vi "getServerCapabilities.vi"(8 "error in (no error)":errorcluster, 11 "IDeviceInfo in":refnum<class "IDeviceInfo.lvclass">) -> (0 "error out":errorcluster, 2 "ServerCapabilty out":refnum<class "IServerCapability.lvclass">[](array[class]), 3 "IDeviceInfo out":refnum<class "IDeviceInfo.lvclass">)   [LabVIEW 2022 SP3, in "openDAQ.lvlib" / "IBaseObject.lvlib" / "IPropertyObject.lvlib" / "IDeviceInfo.lvlib" / "IDeviceInfo.lvclass"]
uses:
  <instrlib>/openDAQ/Public/Classes/IDeviceInfo/IDeviceInfo.lvclass
  <instrlib>/openDAQ/Public/Classes/IDeviceInfo/IDeviceInfo.lvclass/IDeviceInfo.ctl
  <instrlib>/openDAQ/Public/Classes/daqCoreTypes/IList/IList.lvclass
  <instrlib>/openDAQ/Public/Classes/daqCoreTypes/IList/Polymorphic/getList/getServerCapabilityList.vi
  <instrlib>/openDAQ/Binaries/Windows/x86/copendaq32.dll
  <instrlib>/openDAQ/Public/Classes/IServerCapability/IServerCapability.lvclass
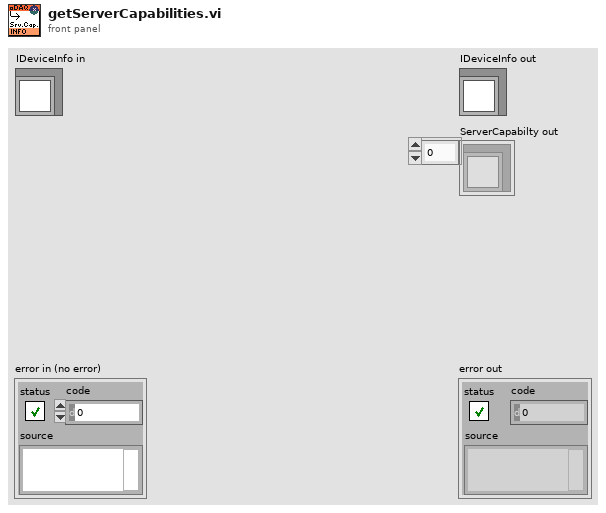
[diagram p1: front panel]
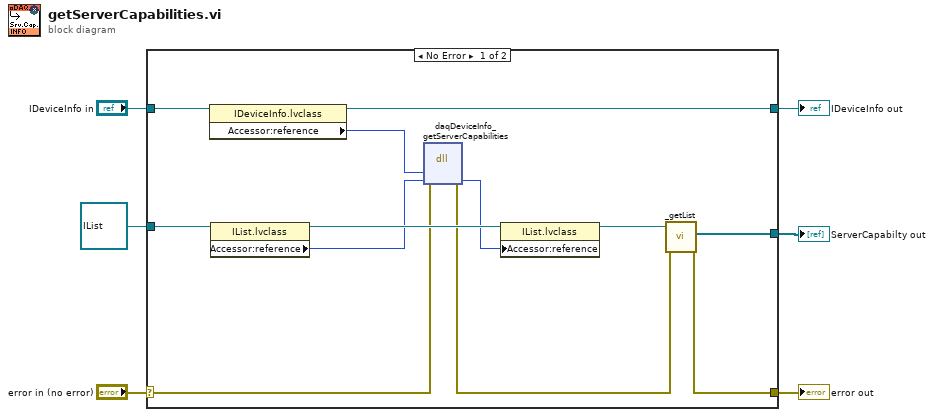
[diagram p0: block diagram]
diagram:
  n1 = case shown="No Error" "error in (no error)" {
    selector: "error in (no error)" -> [w11 w20]
    tunnel: [w7 w20] -> w5
    tunnel: [w15 w19] -> w3
    tunnel: "IDeviceInfo in" -> [w17 w19]
    tunnel: refnum<class "IList.lvclass"> refnum -> [w12 _]
    tunnel: [w9 _] -> w1
    frame No Error {
      n2 = property class="IDeviceInfo.lvclass"(reference=w17) -> (reference out=w15:refnum<class "IDeviceInfo.lvclass">, "Accessor:reference"=w16:i64)  [unwired: 1 in, 1 out]
      n3 = property class="IList.lvclass"(reference=w12) -> (reference out=w18:refnum<class "IList.lvclass">, "Accessor:reference"=w14:i64)  [unwired: 1 in, 1 out]
      n4 = dll-call lib="C:/Program Files (x86)/National Instruments/LabVIEW 2022/instr.lib/openDAQ/Binaries/Windows/x86/copendaq*.*" fn="daqDeviceInfo_getServerCapabilities"(error in=w11, "deviceInfo"=w16, "serverCapability"=w14) -> (error out=w8:errorcluster, "serverCapability"=w13:i64)  [unwired: 4 in, 1 out]
      n5 = property class="IList.lvclass"(reference=w18, "Accessor:reference"=w13) -> (reference out=w10:refnum<class "IList.lvclass">)  [unwired: 1 in, 1 out]
      n6 = call-poly <instrlib>:"_getList.vi"("error in (no error)"=w8, "IList in"=w10) -> ("error out"=w7:errorcluster, "devices out"=w9:refnum<class "IServerCapability.lvclass">[])  [unwired: 8 in]
    }
    frame Error {
    }
  }
  "error out" <- w5
  "IDeviceInfo out" <- w3
  "ServerCapabilty out" <- w1
